vi "New Toggalbe SideMenu.vi"(8 "Error In":errorcluster) -> (0 "Error Out":errorcluster, 3 "Toggable SideMenu":refnum<class "Toggable SideMenu.lvclass">)   [LabVIEW 2021, in "Appearance Actor.lvlib" / "Toggable SideMenu.lvclass"]
uses:
  Toggable SideMenu.lvclass
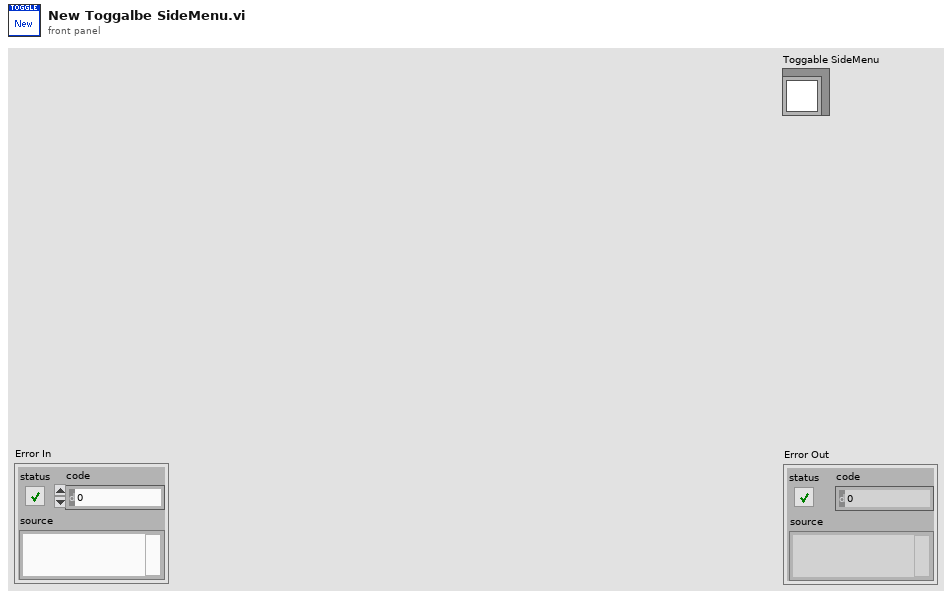
[diagram p1: front panel]
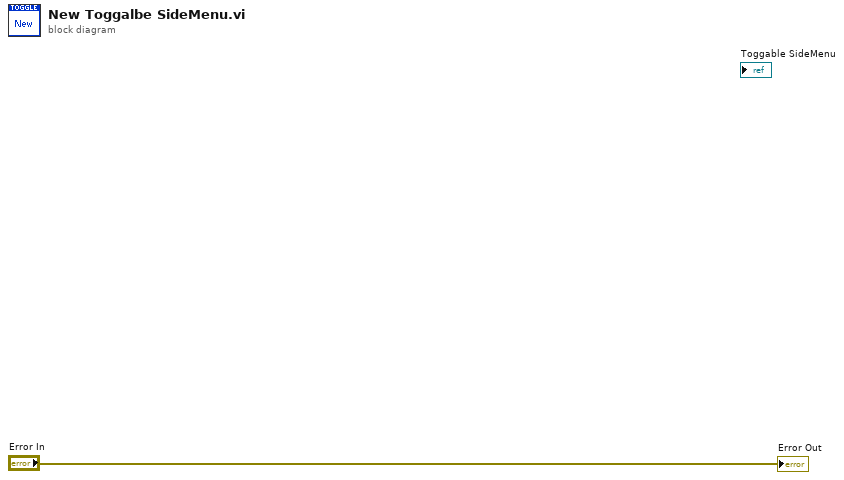
[diagram p0: block diagram]
diagram:
  "Error Out" <- "Error In"
